vi "Dispose.vi"(8 "error in":errorcluster, 11 "ChicagoStyleVeggiePizza":refnum<class "ChicagoStyleVeggiePizza.lvclass">) -> (0 "error out":errorcluster)   [LabVIEW 2020, in "FactoryMethod.lvlib" / "PizzaFactoryMethod.lvlib" / "ChicagoStyleVeggiePizza.lvclass"]
uses:
  ChicagoStyleVeggiePizza.lvclass
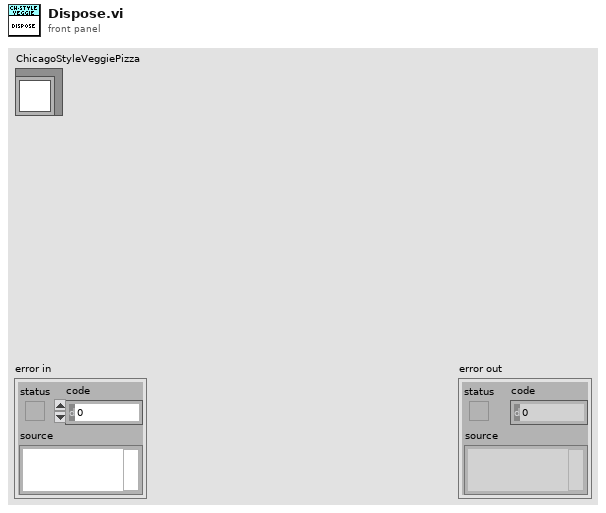
[diagram p1: front panel]
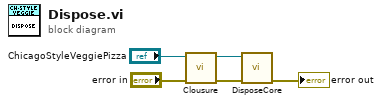
[diagram p0: block diagram]
diagram:
  n1 = call-dynamic "Clousure.vi"("error in"="error in", "ChicagoStyleVeggiePizza"="ChicagoStyleVeggiePizza") -> ("error out"=w3:errorcluster, "ChicagoStyleVeggiePizza"=w4:refnum<class "ChicagoStyleVeggiePizza.lvclass">)  [unwired: 8 in]
  n2 = call-dynamic "DisposeCore.vi"("error in (no error)"=w3, "ChicagoStyleVeggiePizza"=w4) -> ("error out"=→"error out":errorcluster)  [unwired: 8 in, 1 out]
